vi "GetHeadPropertiesInConfigDict.vi"(8 "error in (no error)":errorcluster, 10 "#attributes.HeadNumber":u8, 11 "TopLevel in":refnum<class "TopLevel.lvclass">) -> (0 "error out":errorcluster, 2 "HeadProperties":T1, 3 "TopLevel out":refnum<class "TopLevel.lvclass">)   [LabVIEW 2022 SP3, in "TopLevel.lvclass"]
uses:
  TopLevel.lvclass
  DLP2/DataTypes/DLP2_PrinterHeadProperties.ctl
  Common/Controls/DLPConfig)Init_HeadPropertyAttr--Cluster.ctl
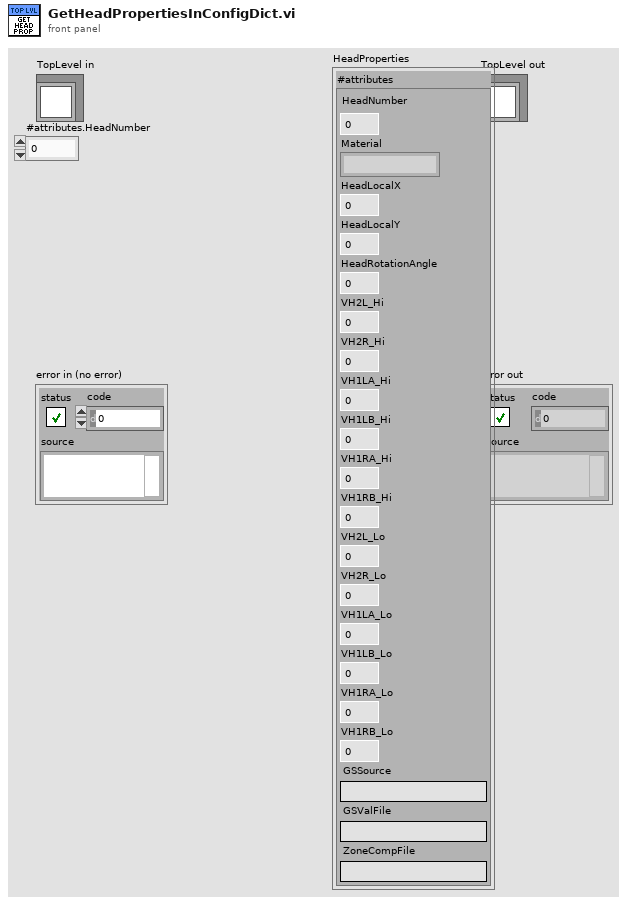
[diagram p1: front panel]
types:
  T1 = typedef "DLP2_PrinterHeadProperties.ctl" = cluster{"#attributes":T2}
  T2 = typedef "DLPConfig)Init_HeadPropertyAttr--Cluster.ctl" = cluster{"HeadNumber":u8, "Material":string, "HeadLocalX":dbl, "HeadLocalY":dbl, "HeadRotationAngle":dbl, "VH2L_Hi":dbl, "VH2R_Hi":dbl, "VH1LA_Hi":dbl, "VH1LB_Hi":dbl, "VH1RA_Hi":dbl, "VH1RB_Hi":dbl, "VH2L_Lo":dbl, "VH2R_Lo":dbl, "VH1LA_Lo":dbl, "VH1LB_Lo":dbl, "VH1RA_Lo":dbl, "VH1RB_Lo":dbl, "GSSource":string, "GSValFile":string, "ZoneCompFile":string}
  T3 = typedef "TD Dynamic CVT DVR--ref.ctl" = refnum<data-value>
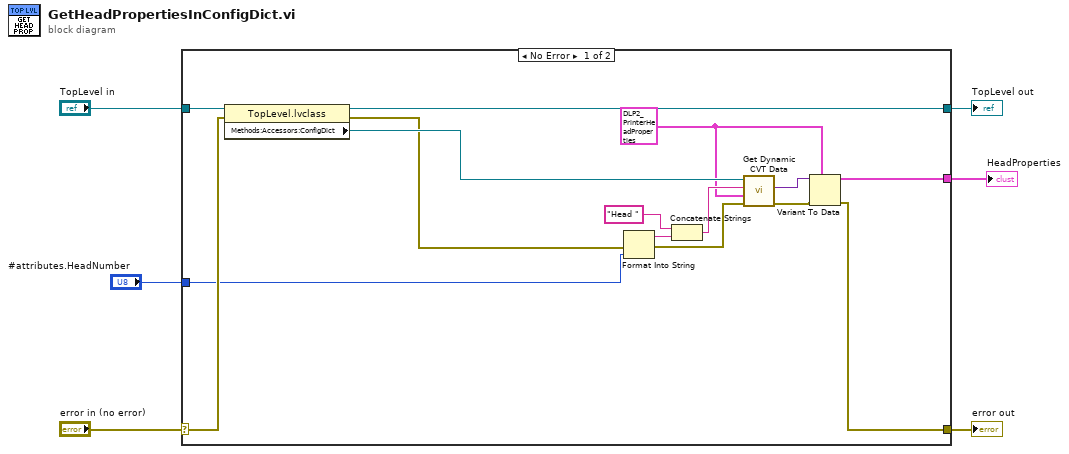
[diagram p0: block diagram]
diagram:
  n1 = case shown="No Error" "error in (no error)" {
    selector: "error in (no error)" -> [w17 w23]
    tunnel: [w9 w23] -> w5
    tunnel: [w19 w22] -> w3
    tunnel: "TopLevel in" -> [w18 w22]
    tunnel: "#attributes.HeadNumber" -> [w16 _]
    tunnel: [w7 _] -> w1
    frame No Error {
      w8 = T1 {"#attributes"={"HeadNumber"=0, "Material"="", "HeadLocalX"=0.0, "HeadLocalY"=0.0, "HeadRotationAngle"=0.0, "VH2L_Hi"=0.0, "VH2R_Hi"=0.0, "VH1LA_Hi"=0.0, "VH1LB_Hi"=0.0, "VH1RA_Hi"=0.0, "VH1RB_Hi"=0.0, "VH2L_Lo"=0.0, "VH2R_Lo"=0.0, "VH1LA_Lo"=0.0, "VH1LB_Lo"=0.0, "VH1RA_Lo"=0.0, "VH1RB_Lo"=0.0, "GSSource"="", "GSValFile"="", "ZoneCompFile"=""}}
      n2 = property class="TopLevel.lvclass"(reference=w18, error in=w17) -> (reference out=w19:refnum<class "TopLevel.lvclass">, error out=w20:errorcluster, "Methods:Accessors:ConfigDict"=w21:T3)
      n3 = Format Into String(error in=w20, w16) -> (resulting string=w14:string, error out=w12:errorcluster)  [unwired: 2 in]
      n4 = Concatenate Strings("Head " ("string"), w14) -> (w13:string)
      n5 = call <vilib>:"Get Dynamic CVT Data.vi"("error in (no error)"=w12, "default value (empty variant)"=w8, "DataName"=w13, "dCVT DVR"=w21) -> ("error out"=w10:errorcluster, "value"=w11:variant)  [unwired: 4 in, 2 out]
      n6 = Variant To Data(error in=w10, type=w8, Variant=w11) -> (data=w7:T1, error out=w9:errorcluster)
    }
    frame Error {
    }
  }
  "error out" <- w5
  "TopLevel out" <- w3
  "HeadProperties" <- w1
